vi "Log Data.vi"(8 "error in (no error)":errorcluster, 10 "Data":waveform(dbl)[](array[waveform]), 11 "Logging Configuration":T1) -> (0 "error out":errorcluster)   [LabVIEW 2016, in "Logging.lvlib"]
doc: "Use the Write To Measurement File Express VI to log data to disk in a LVM file."
uses:
  Logging.lvlib
  Logging Configuration.ctl
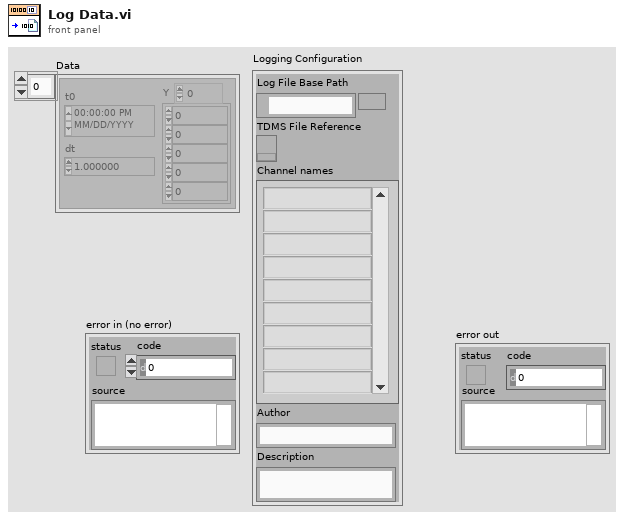
[diagram p1: front panel]
types:
  T1 = typedef "Logging.lvlib/Logging Configuration.ctl" = cluster{"Log File Base Path":path, "TDMS File Reference":refnum<k34>, "Channel names":string[], "Author":string, "Description":string}
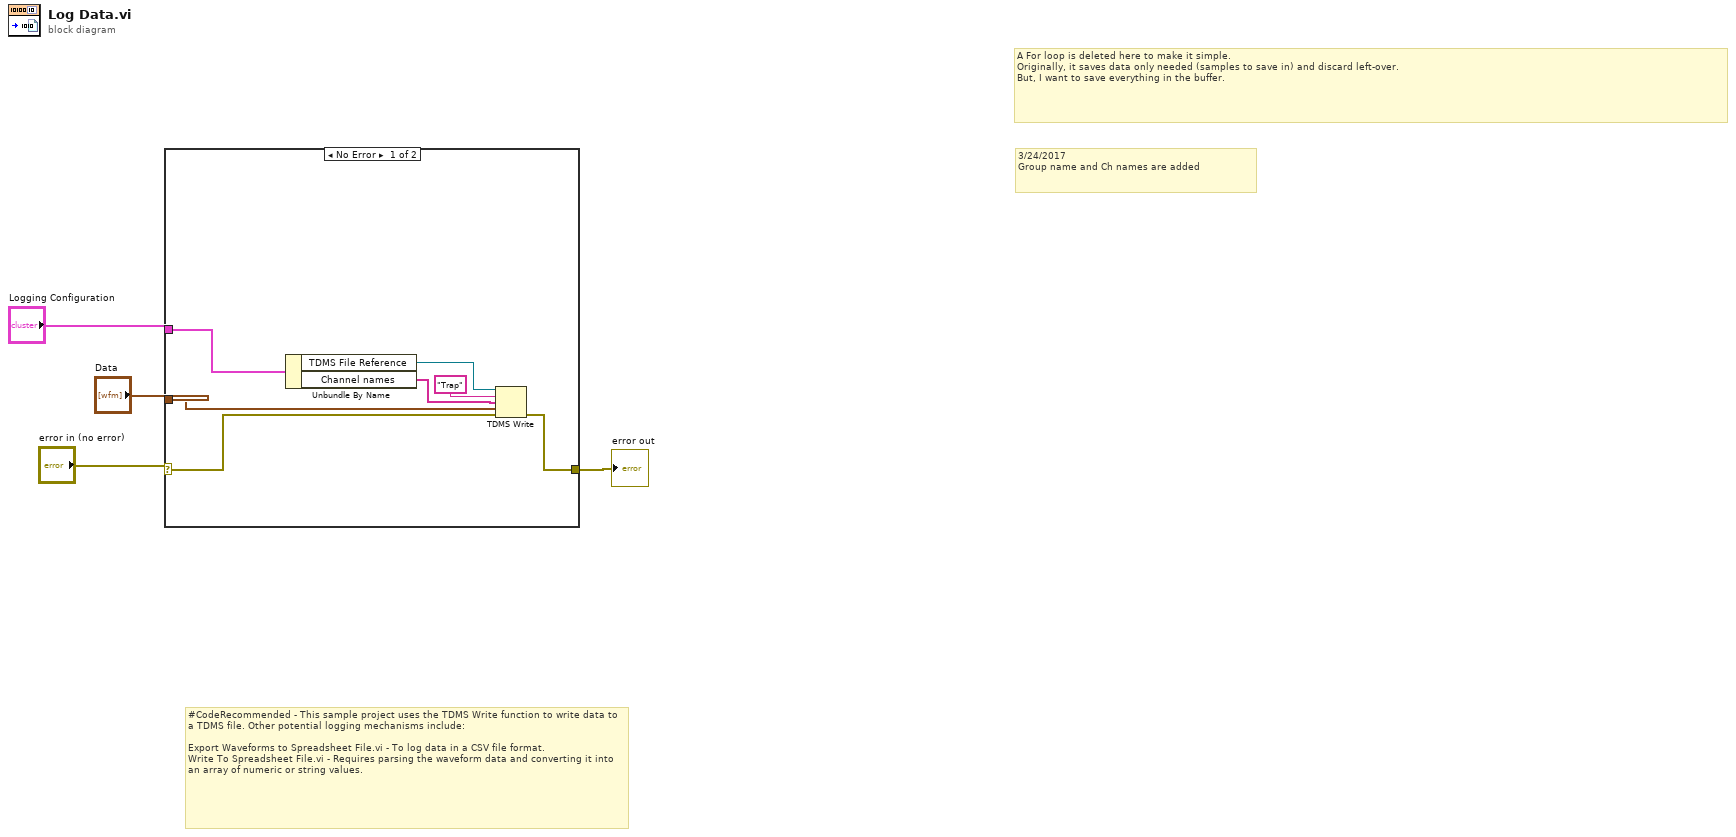
[diagram p0: block diagram]
diagram:
  # "3/24/2017 \nGroup name and Ch names are added"
  # "A For loop is deleted here to make it simple.\nOriginally, it saves data only needed (samples to save in) and discard left-over.\nBut, I want to save everything in the buffer."
  # "#CodeRecommended - This sample project uses the TDMS Write function to write data to a TDMS file. Other potential logging mechanisms include:\n\nExport Waveforms to Spreadsheet File.vi - To log data in a CSV file format.\nWrite To Spreadsheet File.vi - Requires parsing the waveform data and converting it into an array of numeric or string values."
  n1 = case shown="No Error" "error in (no error)" {
    selector: "error in (no error)" -> [w9 w12]
    tunnel: "Logging Configuration" -> [w11 _]
    tunnel: "Data" -> [w8 _]
    tunnel: [w10 w12] -> w3
    frame No Error {
      n2 = Unbundle By Name(w11) -> ("TDMS File Reference"=w7:refnum<k34>, "Channel names"=w6:string[])
      n3 = TDMS Write(0:w7, 5:"Trap" ("group name in (Untitled)"), 7:w6, 9:w8, 11:w9) -> (15:w10:errorcluster)  [unwired: 1 in, 3 out]
    }
    frame Error {
    }
  }
  "error out" <- w3
